vi "Table_UI.vi"(5 "Sort Type":enum16{"numerical", "hex", "string"}(ring), 7 "Sort by":u16(ring) items=["Packet_Number", "Timestamp", "Source", "Destination", "Protocol", "Length", "Data"], 8 "Table Control":refnum<vi>, 9 "Prefiltered Data":string[][](array[string])=array1500x7[10500 elements], 10 "Filter String":string="Protocol == UDP AND Length > 0.7 OR Source == 192.168.1.1", 11 "Headers":string[](array[string])=["Packet Number", "Timestamp", "Source", "Destination", "Protocol", "Length", "Data"]) -> (3 "Table Control":string[][](table))   [LabVIEW 2025, in "Table_Filtering.lvlib"]
uses:
  Table_Filtering.lvlib
panel:
  in  "error in":errorcluster
  out "Error Out":errorcluster
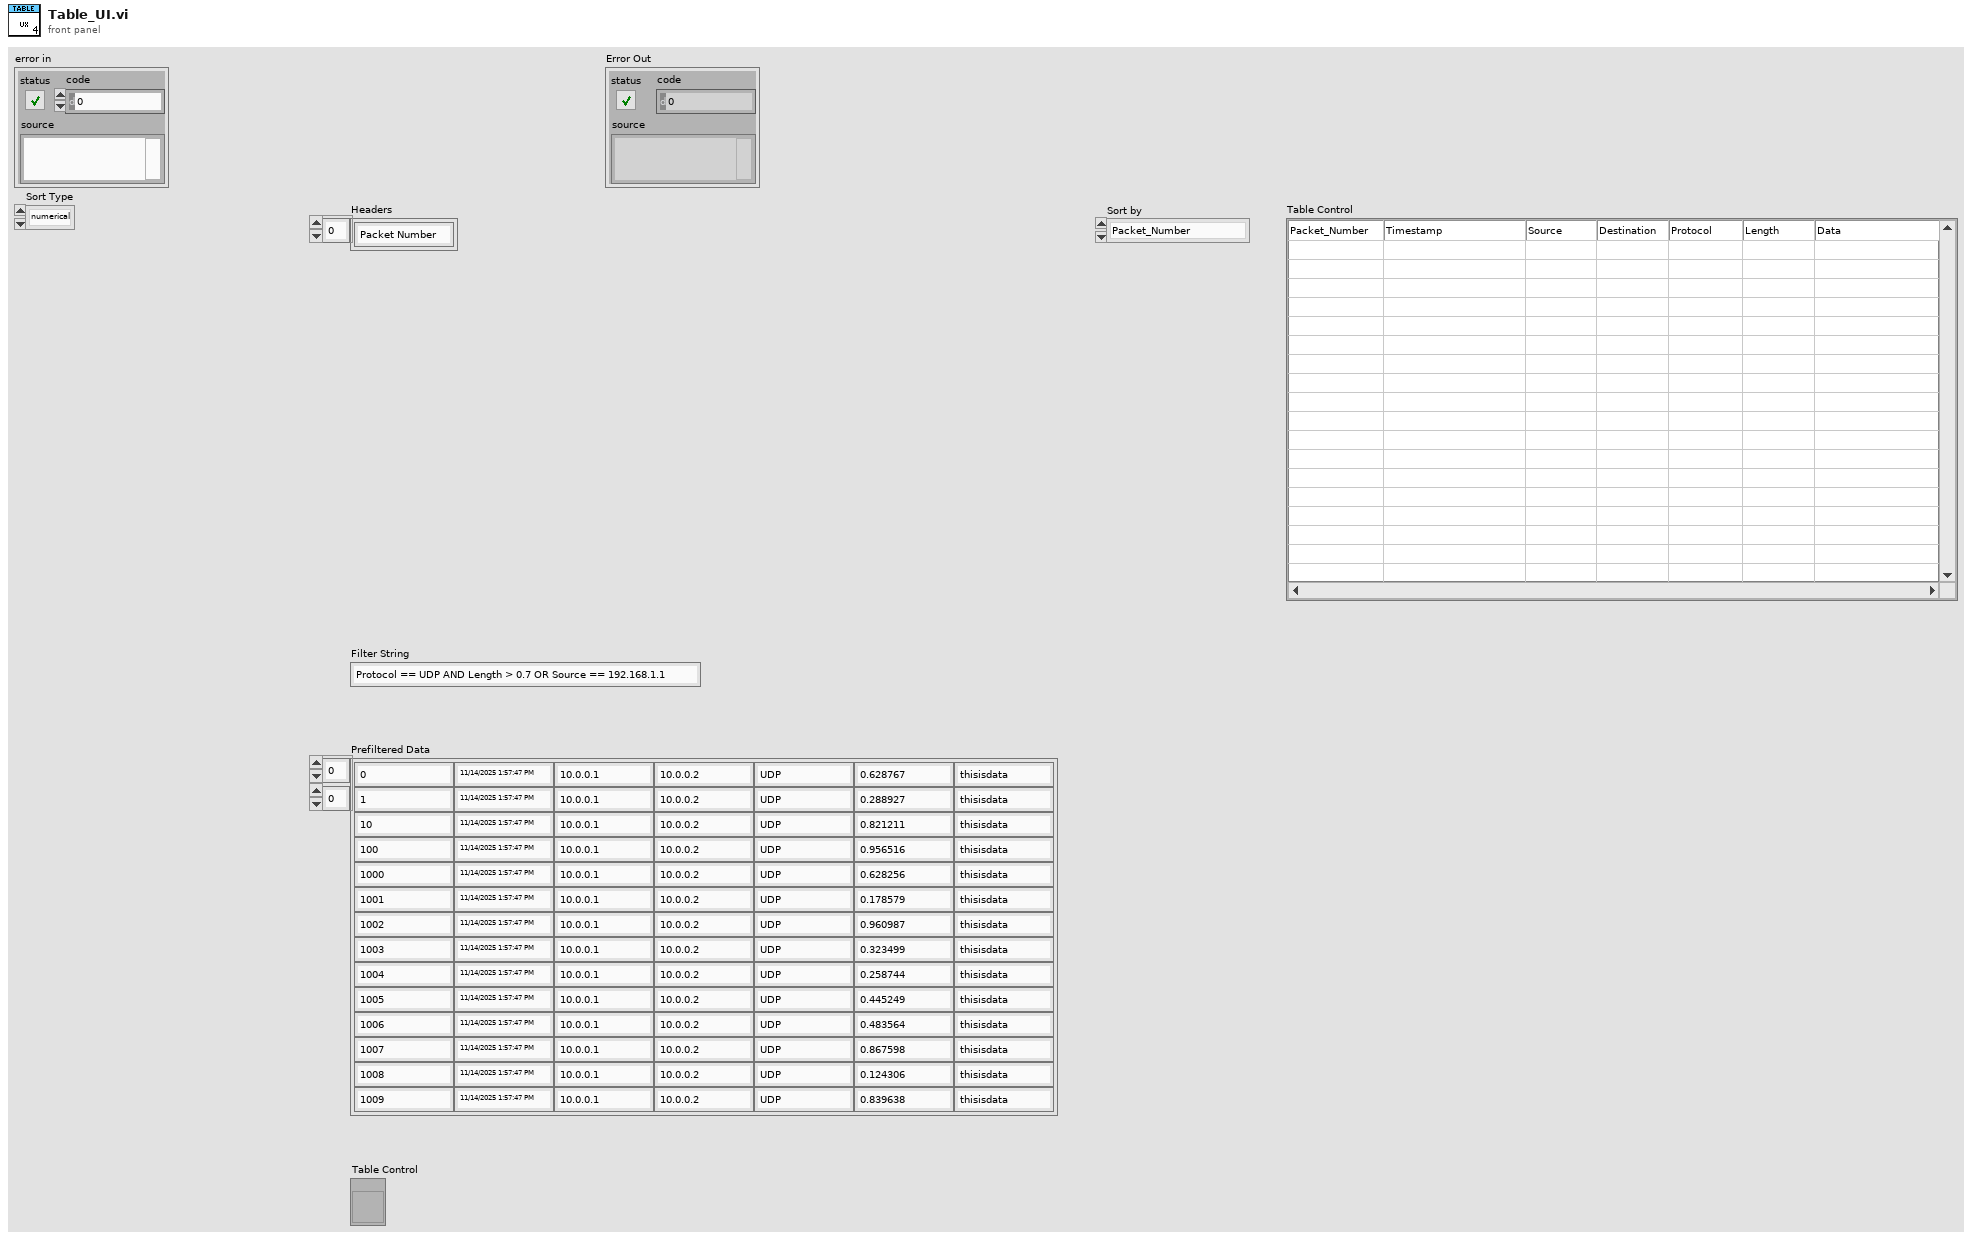
[diagram p1: front panel]
types:
  T1 = cluster{"FIELD":string, "OPERATOR":string, "VALUE":string}[]
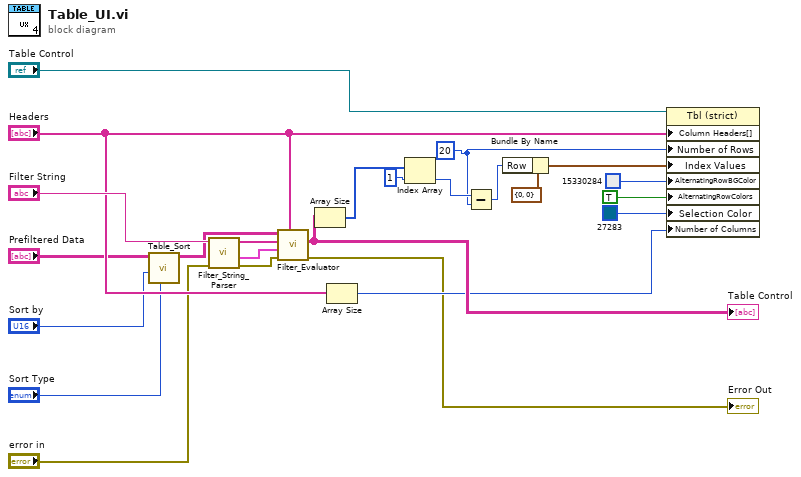
[diagram p0: block diagram]
diagram:
  w14 = 20 ("y")
  n1 = call "Table_Sort.vi"("Sort Type"="Sort Type", "Sort by"="Sort by", "Unsorted Data"="Prefiltered Data") -> ("Sorted data"=w2:string[][])  [unwired: 8 in]
  n2 = call "Filter_String_Parser.vi"("error in"="error in", "Filter String"="Filter String") -> ("error constant"=w7:errorcluster, "Comparators"=w23:T1, "Boolean Connectors"=w22:string[])  [unwired: 7 in]
  n3 = call "Filter_Evaluator.vi"("Headers"="Headers", "Error"=w7, "Comparators"=w23, "Boolean Connectors"=w22, "Prefiltered Data"=w2) -> ("Error Out"=→"Error Out":errorcluster, "Filtered Array"=w15:string[][])  [unwired: 4 in, 1 out]
  "Table Control" <- w15
  n4 = Array Size(array=w15) -> (size(s)=w21:i32[])
  n5 = Array Size(array="Headers") -> (size(s)=w12:i32)
  n6 = Index Array(array=w21, index=1) -> (element=w20:i32)
  n7 = Subtract(x=w20, y=w14) -> (x-y=w19:i32)
  n8 = Bundle By Name(cluster=cluster{"Row":u32, "Column":u32} {"Row"=0, "Column"=0} ("Index Values"), "Row"=w19) -> (w16:cluster{"Row":u32, "Column":u32})
  n9 = property on="Property Node" class="Tbl (strict)"(reference="Table Control", "Column Headers[]"="Headers", "Number of Rows"=w14, "Index Values"=w16, "AlternatingRowBGColor"=u32 15330284 ("Alternate Row Background Color"), "AlternatingRowColors"=TRUE ("Alternating Row Colors"), "Selection Color"=u32 27283, "Number of Columns"=w12) -> ()  [unwired: 1 in, 2 out]
